vi "界面UI.vi"() -> ()   [LabVIEW 2016, in "德润DR803L超标留样.lvlib"]
uses:
  <vilib>/Utility/miscctls.llb/LVPointTypeDef.ctl
  <vilib>/Utility/config.llb/NI_LVConfig.lvlib
  <vilib>/ptbypt/NI_PtbyPt.lvlib
panel:
  in  "超标浓度配置":bool
  out "流程中":bool
  in  "停止流程":bool
  in  "启动流程":bool
  in  "时间等比采样":u16=10
  in  "单次采样量":u16=500
  in  "修改门禁密码":bool
  in  "远程复位":bool
  in  "排空当前瓶":bool
  in  "采样方式":enum16{"单采", "双重"}(ring)
  in  "远程留样":bool
  in  "选择留样瓶":bool
  in  "排空留样瓶":bool
  out "采样器状态":T1
  out "Registers":u16[](array[numeric])
  in  "打开串口":bool
  in  "释放串口":bool
  in  "留样模式":T2(ring)=enum."外控留样"
  in  "采样启动":bool
  in  "停止命令":bool
  in  "切换采样器状态":bool
  in  "时间校准":bool
  out "source":string
  out "通讯":bool
  # "只在停止时切换有效"
  # "只在待机时切换有效"
  # "默认：500ml（5-1000）ml （只在停止时写有效）"
  # "只在待机时启动有效"
  # "默认：10min（2-9999）min （只在停止时写有效）"
  # "只在待机时启动有效"
  # "只在待机时启动有效"
  # "德润DR803L超标留样"
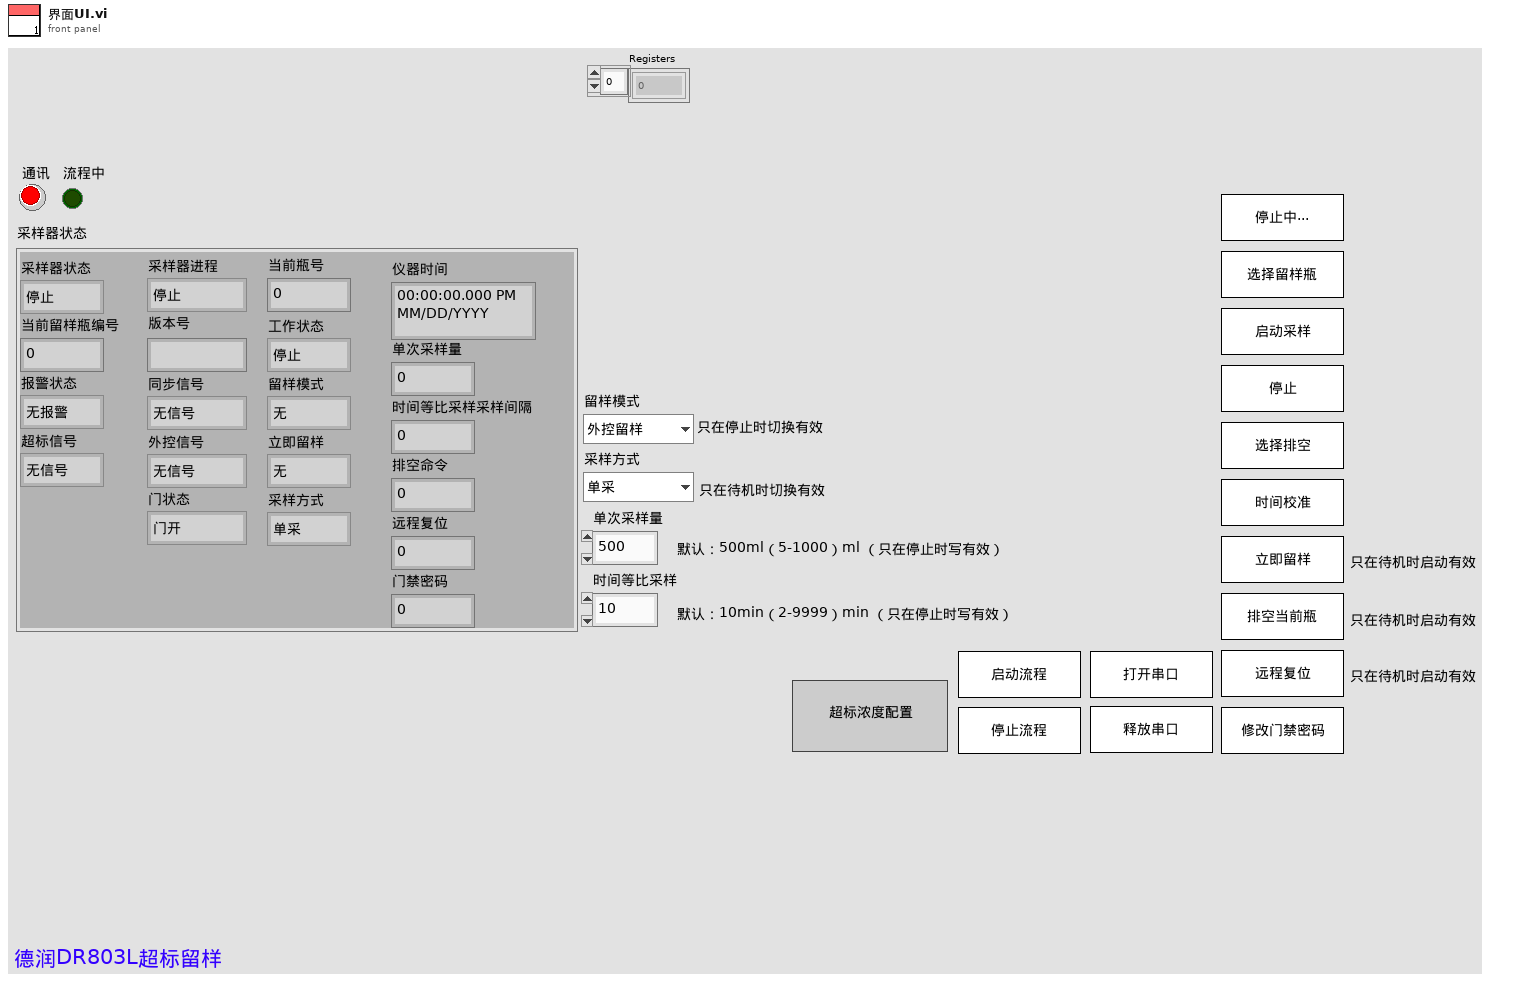
[diagram p1: front panel]
types:
  T1 = cluster{"采样器状态":enum16{"停止", "运行"}, "当前留样瓶编号":u16, "报警状态":enum16{"无报警", "缺水报警"}, "超标信号":enum16{"无信号", "超标信号"}, "采样器进程":enum16{"停止", "待机", "定位校正", "移除瓶盖", "采样瓶排空", "管路润洗", "管存", "进样", "瓶盖密封", "管路排空", "调整采样位置", "采样结束", "采样瓶润洗", "瓶润洗排空"}, "版本号":string, "同步信号":enum16{"无信号", "同步信号"}, "外控信号":enum16{"无信号", "外控信号"}, "门状态":enum16{"门开", "门关"}, "当前瓶号":u16, "工作状态":enum16{"停止", "采样中"}, "留样模式":enum16{"无", "定时留样", "时间等比例", "超标留样", "同步留样", "外控留样"}, "立即留样":enum16{"无", "远程留样"}, "采样方式":enum16{"单采", "双重"}, "仪器时间":timestamp, "单次采样量":u16, "时间等比采样采样间隔":u16, "排空命令":u16, "远程复位":u16, "门禁密码":u16}
  T2 = enum16{"无", "定时留样", "时间等比例", "超标留样", "同步留样", "外控留样"}
  T3 = cluster{"STEP":enum16{"open", "read", "write", "write single", "close"}, "starting address":u16, "value":u16}
  T4 = typedef "LVPointTypeDef.ctl" = cluster{"Horizontal":i16, "Vertical":i16}
  T5 = typedef "NI_LVConfig.lvlib/Config Data RefNum.ctl" = refnum<k1>
  T6 = enum16{"open", "read", "write", "write single", "close"}
  T7 = cluster{"氨氮超标浓度":dbl, "总磷超标浓度":dbl, "总氮超标浓度":dbl, "CODMn超标浓度":dbl, "CODCr超标浓度":dbl}
  T8 = typedef "LVDateTimeRec.ctl" = cluster{"秒数的小数部分":dbl, "秒":i32, "分":i32, "时":i32, "日":i32, "月":i32, "年":i32, "天数（周）":i32, "天数（年）":i32, "DST":i32}
  T9 = enum32{"Bad", "Idle", "Run top level", "Running"}
  T10 = cluster{"确定":bool, "氨氮超标浓度":dbl, "总磷超标浓度":dbl, "总氮超标浓度":dbl, "CODMn超标浓度":dbl, "CODCr超标浓度":dbl}
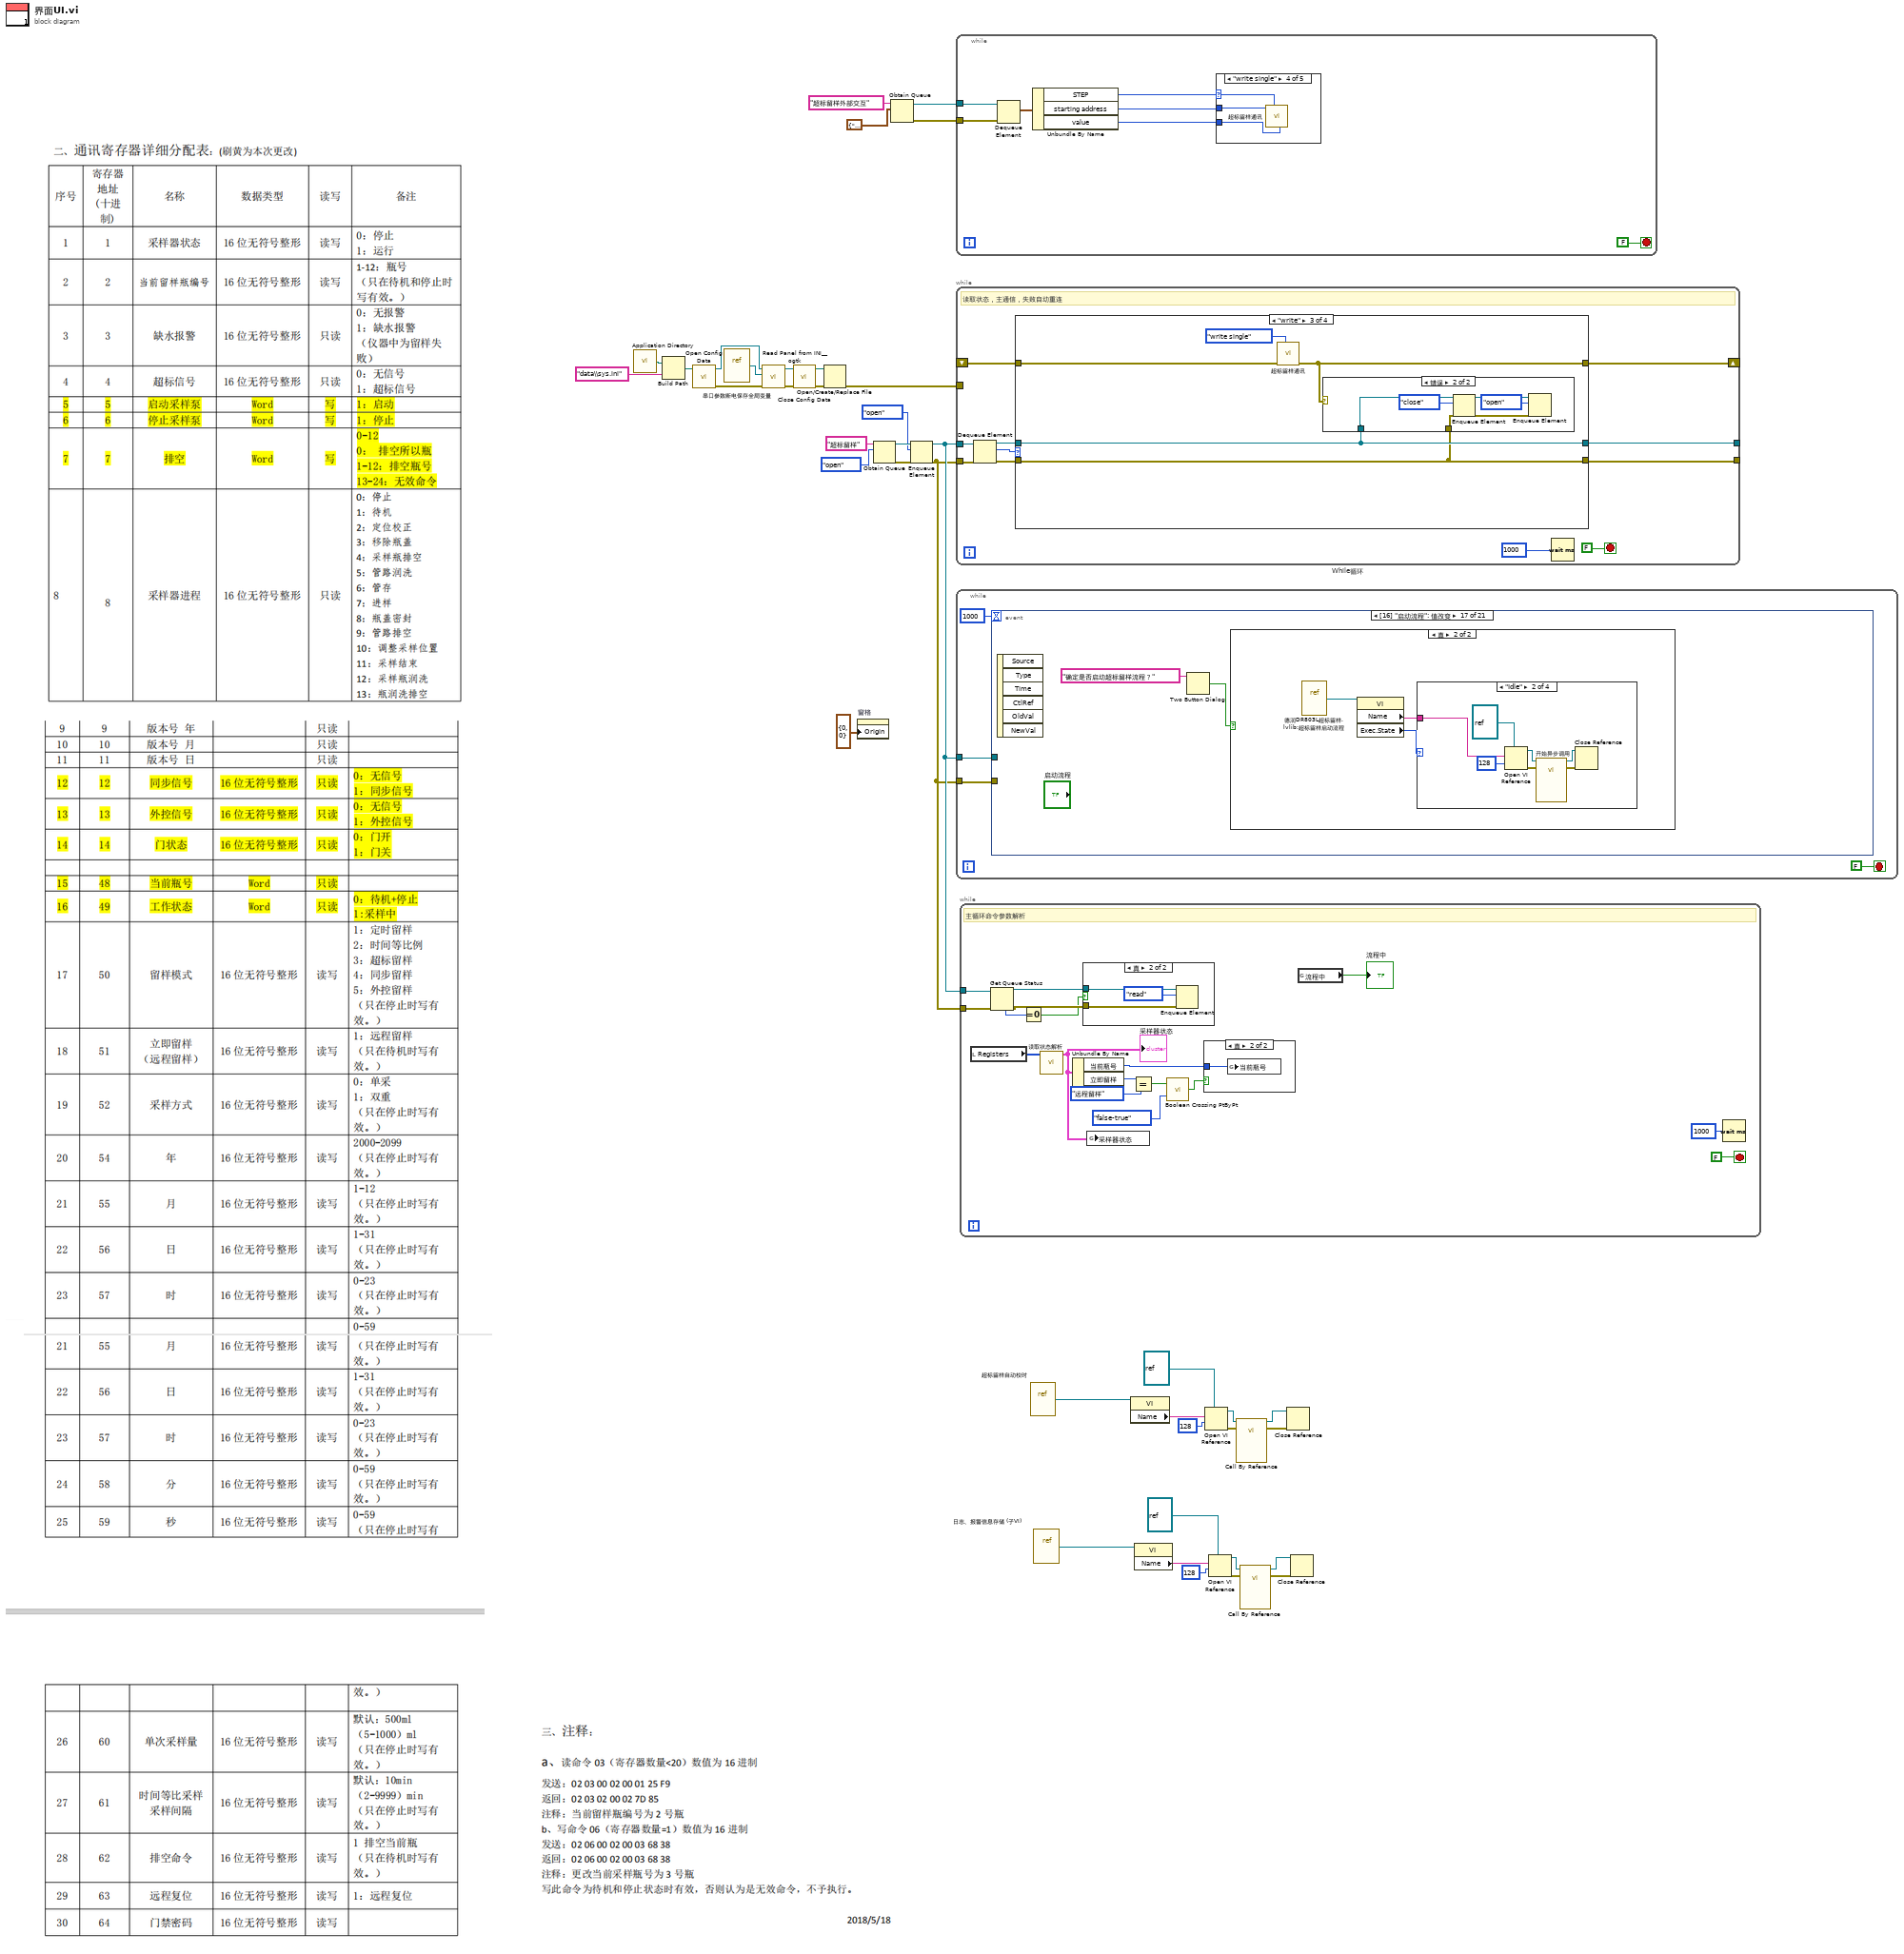
[diagram p0: block diagram]
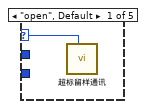
[diagram p2: hidden frame]
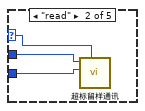
[diagram p3: hidden frame]
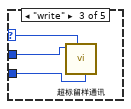
[diagram p4: hidden frame]
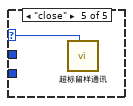
[diagram p5: hidden frame]
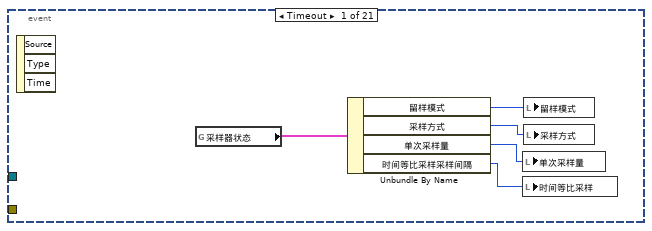
[diagram p6: hidden frame]
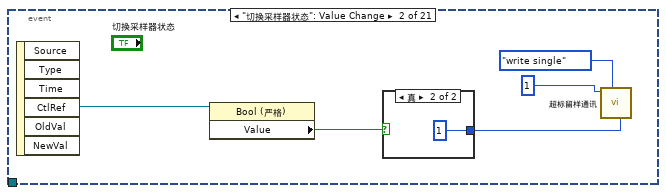
[diagram p7: hidden frame]
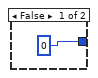
[diagram p8: hidden frame]
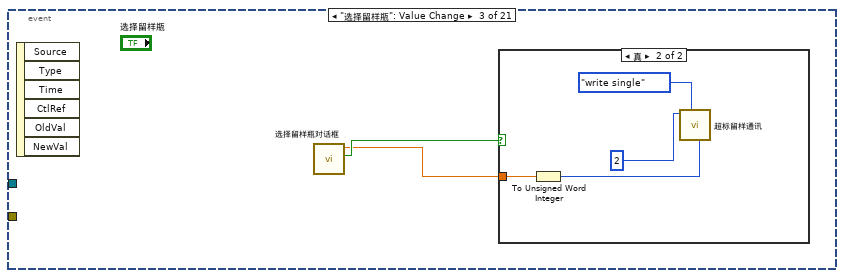
[diagram p9: hidden frame]
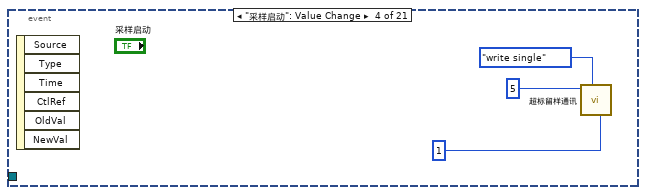
[diagram p11: hidden frame]
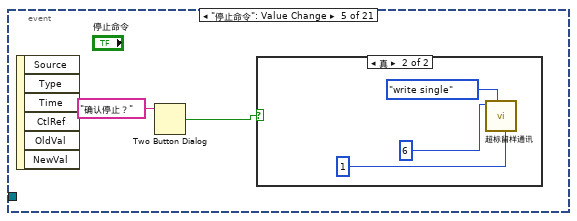
[diagram p12: hidden frame]
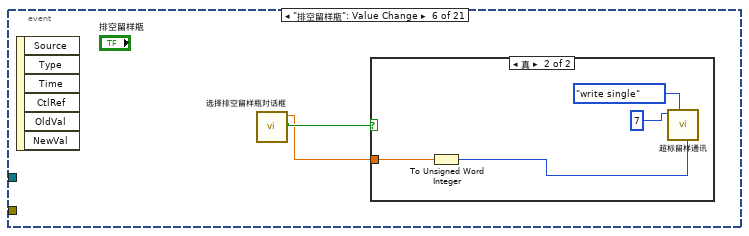
[diagram p14: hidden frame]
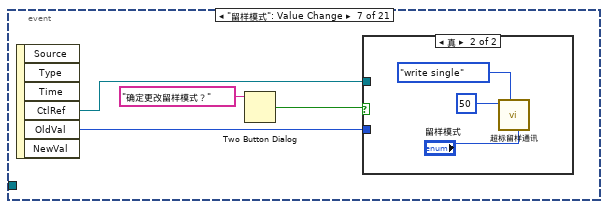
[diagram p16: hidden frame]
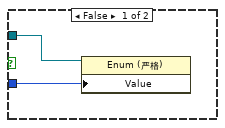
[diagram p17: hidden frame]
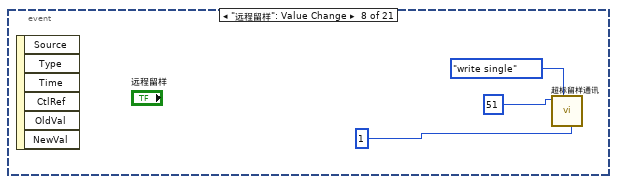
[diagram p18: hidden frame]
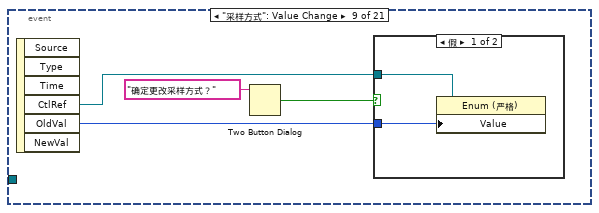
[diagram p19: hidden frame]
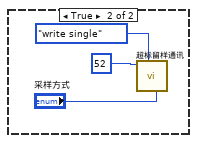
[diagram p20: hidden frame]
diagram:
  n1 = call <vilib>:"Application Directory.vi"() -> ("Application Directory"=w31:path)
  n2 = Build Path(base path=w31, name or relative path="data\\sys.ini" ("名称或相对路径")) -> (appended path=w29:path)
  n3 = call <vilib>:"Open Config Data.vi"("configuration file path"=w29) -> ("error out"=w25:errorcluster, "refnum"=w28:T5)  [unwired: 8 in, 1 out]
  n4 = vi-ref "串口参数断电保存全局变量.vi"() -> (w27:refnum<vi>)
  n5 = call <userlib>:"Read Panel from INI__ogtk.vi"("error in (no error)"=w25, "VI ref"=w27, "refnum"=w28) -> ("error out"=w24:errorcluster, "refnum out"=w26:T5)  [unwired: 7 in]
  n6 = call <vilib>:"Close Config Data.vi"("error in (no error)"=w24, "refnum"=w26) -> ("error out"=w23:errorcluster, "file path"=w22:path)  [unwired: 8 in]
  n7 = Open/Create/Replace File(file path (use dialog)=w22, error in=w23) -> (error out=w21:errorcluster)  [unwired: 4 in, 2 out]
  n8 = property on="窗格" class="Pane"("Origin"=T4 {"Horizontal"=0, "Vertical"=0} ("原点")) -> ()  [unwired: 2 in, 2 out]
  n9 = Obtain Queue(name (unnamed)="超标留样" ("名称（未命名）"), element data type=enum16{"open", "read", "write", "close"}."open") -> (queue out=w37:refnum<queue>, error out=w36:errorcluster)  [unwired: 3 in, 1 out]
  n10 = Obtain Queue(name (unnamed)="超标留样外部交互" ("名称（未命名）"), element data type=T3 {"STEP"=enum."write single", "starting address"=0, "value"=0}) -> (queue out=w18:refnum<queue>, error out=w17:errorcluster)  [unwired: 3 in, 1 out]
  n11 = Enqueue Element(queue=w37, element=enum16{"open", "read", "write", "close"}."open", error in (no error)=w36) -> (queue out=w34:refnum<queue>, error out=w33:errorcluster)  [unwired: 1 in, 1 out]
  n12 = while {
    tunnel: w34 -> [w42]
    tunnel: w33 -> [w41]
    stop <- FALSE stop-if-true
    n13 = event shown="[16] \"启动流程\": 值改变" {
      selector: _ -> [_ _ _ _ _ _ _ _ _ _ _ _ _ _ _ _ _ _ _ _ _]
      dyn-events: _ -> [_ _ _ _ _ _ _ _ _ _ _ _ _ _ _ _ _ _ _ _ _]
      timeout: 1000 -> [_ _ _ _ _ _ _ _ _ _ _ _ _ _ _ _ _ _ _ _ _]
      tunnel: w42 -> [_ _ _ _ _ _ _ _ _ _ _ _ _ _ _ _ _ _ w171 w177 _]
      tunnel: w41 -> [_ _ _ _ _ _ _ _ _ _ _ _ _ _ _ _ _ _ w170 w176 _]
      event Timeout {
        n14 = event-data() -> ()  [unwired: 1 in, 3 out]
        n15 = global read "超标留样全局.vi" "采样器状态"() -> (w44:T1)
        n16 = Unbundle By Name(w44) -> ("留样模式"=w48:T2, "采样方式"=w45:enum16{"单采", "双重"}, "单次采样量"=w46:u16, "时间等比采样采样间隔"=w47:u16)
        n17 = local write "单次采样量"(w46) -> ()
        n18 = local write "时间等比采样"(w47) -> ()
        n19 = local write "留样模式"(w48) -> ()
        n20 = local write "采样方式"(w45) -> ()
      }
      event "切换采样器状态": Value Change {
        n21 = event-data() -> ("CtlRef"=w53:refnum<vi>)  [unwired: 1 in, 5 out]
        n22 = property class="Bool (严格)"(reference=w53) -> ("Value"=w52:bool)  [unwired: 1 in, 2 out]
        n23 = case shown="真" w52 {
          tunnel: [u16 0 ("索引") u16 1 ("索引")] -> w49
          frame False {
          }
          frame True {
          }
        }
        n24 = call "超标留样通讯.vi"("value"=w49, "STEP"=T6."write single", "starting address"=1 ("索引")) -> ()  [unwired: 6 in, 3 out]
      }
      event "选择留样瓶": Value Change {
        n25 = event-data() -> ()  [unwired: 1 in, 6 out]
        n26 = call "选择留样瓶对话框.vi"() -> ("布尔"=w57:bool, "选择留样瓶"=w56:dbl)  [unwired: 10 in]
        n27 = case shown="真" w57 {
          tunnel: w56 -> [_ w58]
          frame False {
          }
          frame True {
            n28 = To Unsigned Word Integer(number=w58) -> (unsigned 16bit integer=w59:u16)
            n29 = call "超标留样通讯.vi"("value"=w59, "STEP"=T6."write single", "starting address"=2 ("索引")) -> ()  [unwired: 6 in, 3 out]
          }
        }
      }
      event "采样启动": Value Change {
        n30 = event-data() -> ()  [unwired: 1 in, 6 out]
        n31 = call "超标留样通讯.vi"("value"=u16 1 ("新元素/子数组"), "STEP"=T6."write single", "starting address"=5 ("索引")) -> ()  [unwired: 6 in, 3 out]
      }
      event "停止命令": Value Change {
        n32 = event-data() -> ()  [unwired: 1 in, 6 out]
        n33 = Two Button Dialog(message="确认停止？" ("消息")) -> (T button?=w65:bool)  [unwired: 2 in]
        n34 = case shown="真" w65 {
          frame False {
          }
          frame True {
            n35 = call "超标留样通讯.vi"("value"=u16 1 ("新元素/子数组"), "STEP"=T6."write single", "starting address"=6 ("索引")) -> ()  [unwired: 6 in, 3 out]
          }
        }
      }
      event "排空留样瓶": Value Change {
        n36 = event-data() -> ()  [unwired: 1 in, 6 out]
        n37 = call "选择排空留样瓶对话框.vi"() -> ("布尔"=w71:bool, "选择留样瓶"=w70:dbl)  [unwired: 10 in]
        n38 = case shown="真" w71 {
          tunnel: w70 -> [_ w75]
          frame False {
          }
          frame True {
            n39 = To Unsigned Word Integer(number=w75) -> (unsigned 16bit integer=w72:u16)
            n40 = call "超标留样通讯.vi"("value"=w72, "STEP"=T6."write single", "starting address"=7 ("索引")) -> ()  [unwired: 6 in, 3 out]
          }
        }
      }
      event "留样模式": Value Change {
        n41 = event-data() -> ("CtlRef"=w76:refnum<vi>, "OldVal"=w77:T2)  [unwired: 1 in, 4 out]
        n42 = Two Button Dialog(message="确定更改留样模式？" ("消息")) -> (T button?=w78:bool)  [unwired: 2 in]
        n43 = case shown="真" w78 {
          tunnel: w77 -> [w80 _]
          tunnel: w76 -> [w81 _]
          frame False {
            n44 = property class="Enum (严格)"(reference=w81, "Value"=w80) -> ()  [unwired: 1 in, 2 out]
          }
          frame True {
            n45 = call "超标留样通讯.vi"("value"="留样模式", "STEP"=T6."write single", "starting address"=50 ("索引")) -> ()  [unwired: 6 in, 3 out]
          }
        }
      }
      event "远程留样": Value Change {
        n46 = event-data() -> ()  [unwired: 1 in, 6 out]
        n47 = call "超标留样通讯.vi"("value"=u16 1 ("新元素/子数组"), "STEP"=T6."write single", "starting address"=51 ("索引")) -> ()  [unwired: 6 in, 3 out]
      }
      event "采样方式": Value Change {
        n48 = event-data() -> ("CtlRef"=w89:refnum<vi>, "OldVal"=w88:enum16{"单采", "双重"})  [unwired: 1 in, 4 out]
        n49 = Two Button Dialog(message="确定更改采样方式？" ("消息")) -> (T button?=w90:bool)  [unwired: 2 in]
        n50 = case shown="假" w90 {
          tunnel: w89 -> [w93 _]
          tunnel: w88 -> [w92 _]
          frame False {
            n51 = property class="Enum (严格)"(reference=w93, "Value"=w92) -> ()  [unwired: 1 in, 2 out]
          }
          frame True {
            n52 = call "超标留样通讯.vi"("value"="采样方式", "STEP"=T6."write single", "starting address"=52 ("索引")) -> ()  [unwired: 6 in, 3 out]
          }
        }
      }
      event "时间校准": Value Change {
        n53 = event-data() -> ()  [unwired: 1 in, 6 out]
        n54 = Get Date/Time In Seconds() -> (seconds since 1Jan1904=w109:timestamp)
        n55 = Seconds To Date/Time(time stamp (now)=w109) -> (date time rec=w108:T8)  [unwired: 1 in]
        n56 = Unbundle By Name(w108) -> ("年"=w105:i32, "月"=w104:i32, "日"=w103:i32, "时"=w102:i32, "分"=w101:i32, "秒"=w100:i32)
        n57 = Build Array(w105, w104, w103, w102, w101, w100) -> (w99:i32[])
        n58 = Insert Into Array(array=u16[] [] ("values"), new element=w99) -> (w106:u16[])  [unwired: 1 in]
        n59 = call "超标留样通讯.vi"("STEP"=T6."write", "values"=w106, "starting address"=54 ("索引")) -> ()  [unwired: 6 in, 3 out]
      }
      event "单次采样量", "时间等比采样": Mouse Down {
        n60 = event-data() -> ("CtlRef"=w113:refnum<vi>)  [unwired: 1 in, 7 out]
        n61 = property class="DigNum (严格)"(reference=w113) -> (reference out=w112:refnum<vi>, "Value"=w111:u16)  [unwired: 1 in, 1 out]
        n62 = call "数字键盘.vi"("OldNumber"=w111) -> ("NewNumber"=w110:sgl)
        n63 = property class="DigNum (严格)"(reference=w112, "Val(Sgnl)"=w110) -> ()  [unwired: 1 in, 2 out]
      }
      event "单次采样量": Value Change {
        n64 = event-data() -> ()  [unwired: 1 in, 6 out]
        n65 = call "超标留样通讯.vi"("value"="单次采样量", "STEP"=T6."write single", "starting address"=60 ("索引")) -> ()  [unwired: 6 in, 3 out]
      }
      event "时间等比采样": Value Change {
        n66 = event-data() -> ()  [unwired: 1 in, 6 out]
        n67 = call "超标留样通讯.vi"("value"="时间等比采样", "STEP"=T6."write single", "starting address"=61 ("索引")) -> ()  [unwired: 6 in, 3 out]
      }
      event "排空当前瓶": Value Change {
        n68 = event-data() -> ()  [unwired: 1 in, 6 out]
        n69 = Two Button Dialog(message="是否排空当前瓶？" ("消息")) -> (T button?=w120:bool)  [unwired: 2 in]
        n70 = case shown="真" w120 {
          frame False {
          }
          frame True {
            n71 = call "超标留样通讯.vi"("value"=u16 1 ("新元素/子数组"), "STEP"=T6."write single", "starting address"=63 ("索引")) -> ()  [unwired: 6 in, 3 out]
          }
        }
      }
      event "远程复位": Value Change {
        n72 = event-data() -> ()  [unwired: 1 in, 6 out]
        n73 = Two Button Dialog(message="确认复位？" ("消息")) -> (T button?=w125:bool)  [unwired: 2 in]
        n74 = case shown="真" w125 {
          frame False {
          }
          frame True {
            n75 = call "超标留样通讯.vi"("value"=u16 1 ("新元素/子数组"), "STEP"=T6."write single", "starting address"=64 ("索引")) -> ()  [unwired: 6 in, 3 out]
          }
        }
      }
      event "修改门禁密码": Value Change {
        n76 = event-data() -> ()  [unwired: 1 in, 6 out]
        n77 = Two Button Dialog(message="确定修改门禁密码？" ("消息")) -> (T button?=w130:bool)  [unwired: 2 in]
        n78 = case shown="真" w130 {
          frame False {
          }
          frame True {
            n79 = local read "采样器状态"() -> (w133:T1)
            n80 = Unbundle By Name(w133) -> ("门禁密码"=w132:u16)
            n81 = call "数字键盘.vi"("OldNumber"=w132) -> ("NewNumber"=w136:sgl)
            n82 = Less?(x=w136, y=sgl 65535.0) -> (x < y?=w134:bool)
            n83 = case shown="真" w134 {
              tunnel: w136 -> [_ w140]
              frame False {
              }
              frame True {
                n84 = To Unsigned Word Integer(number=w140) -> (unsigned 16bit integer=w137:u16)
                n85 = call "超标留样通讯.vi"("value"=w137, "STEP"=T6."write single", "starting address"=65 ("索引")) -> ()  [unwired: 6 in, 3 out]
              }
            }
          }
        }
      }
      event "启动流程": Value Change {
        n86 = event-data() -> ()  [unwired: 1 in, 6 out]
        n87 = Two Button Dialog(message="确定是否启动超标留样流程？" ("消息")) -> (T button?=w141:bool)  [unwired: 2 in]
        n88 = case shown="真" w141 {
          frame False {
          }
          frame True {
            n89 = vi-ref "德润DR803L超标留样.lvlib:超标留样启动流程.vi"() -> (w143:refnum<vi>)
            n90 = property class="VI"(reference=w143) -> ("Name"=w144:string, "Exec.State"=w145:T9)  [unwired: 1 in, 2 out]
            n91 = case shown="\"Idle\"" w145 {
              tunnel: w144 -> [_ w148 _ _]
              frame "Bad", Default {
              }
              frame "Idle" {
                n92 = Open VI Reference(type specifier VI Refnum (for type only)=refnum<vi> refnum ("类型说明符VI引用句柄（仅用于类型）"), vi path=w148, options=128 ("选项")) -> (vi reference=w152:refnum<vi>, error out=w147:errorcluster)  [unwired: 3 in]
                n93 = call-by-ref "开始异步调用"(reference=w152, error in=w147) -> (reference out=w151:refnum<vi>, error out=w146:errorcluster)  [unwired: 12 in]
                n94 = Close Reference(reference=w151, error in (no error)=w146) -> ()  [unwired: 1 out]
              }
              frame "Run top level" {
              }
              frame "Running" {
              }
            }
          }
        }
      }
      event "停止流程": Value Change {
        n95 = event-data() -> ()  [unwired: 1 in, 6 out]
        n96 = Two Button Dialog(message="确定是否停止超标留样流程并排空当前瓶？" ("消息")) -> (T button?=w153:bool)  [unwired: 2 in]
        n97 = case shown="真" w153 {
          frame False {
          }
          frame True {
            n98 = Obtain Notifier(name (unnamed)="超标留样流程" ("名称（未命名）"), notification data type=FALSE ("采样完成")) -> (notifier out=w166:refnum<notifier>, error out=w165:errorcluster)  [unwired: 2 in, 1 out]
            n99 = Send Notification(notification=TRUE ("通知"), notifier=w166, error in (no error)=w165) -> (notifier out=w163:refnum<notifier>, error out=w162:errorcluster)
            n100 = call "超标留样通讯.vi"("value"=u16 1 ("新元素/子数组"), "STEP"=T6."write single", "starting address"=6 ("索引")) -> ("error out"=w155:errorcluster)  [unwired: 6 in, 2 out]
            n101 = Release Notifier(notifier=w163, error in (no error)=w162) -> ()  [unwired: 1 in, 3 out]
            n102 = call "超标留样通讯.vi"("value"=u16 1 ("新元素/子数组"), "STEP"=T6."write single", "Error in"=w155, "starting address"=63 ("索引")) -> ()  [unwired: 5 in, 3 out]
          }
        }
      }
      event "释放串口": Value Change {
        n103 = event-data() -> ()  [unwired: 1 in, 6 out]
        n104 = Two Button Dialog(message="确认是否释放串口，释放串口将导致通信失败！" ("消息")) -> (T button?=w169:bool)  [unwired: 2 in]
        n105 = case shown="真" w169 {
          tunnel: w171 -> [_ w174]
          tunnel: w170 -> [_ w173]
          frame False {
          }
          frame True {
            n106 = Enqueue Element(queue=w174, element=enum16{"open", "read", "write", "close"}."close" ("元素"), error in (no error)=w173) -> ()  [unwired: 1 in, 3 out]
          }
        }
      }
      event "打开串口": Value Change {
        n107 = event-data() -> ()  [unwired: 1 in, 6 out]
        n108 = global read "串口参数断电保存全局变量.vi" "VISA resource name"() -> (w185:refnum<visa-resource-name>)
        n109 = global read "串口参数断电保存全局变量.vi" "MB通信方式选择"() -> (w186:enum16{"串口", "TCP"})
        n110 = global read "串口参数断电保存全局变量.vi" "PORT"() -> (w183:string)
        n111 = global read "串口参数断电保存全局变量.vi" "IP"() -> (w184:string)
        n112 = call "串口配置.vi"("PORT"=w183, "IP"=w184, "MB通信方式选择"=w186, "请选择串口:"=w185) -> ("PORT 2"=w179:string, "IP 2"=w180:string, "确认 2"=w182:bool, "VISA资源名称 2"=w181:refnum<visa-resource-name>, "MB通信方式选择 2"=w178:enum16{"串口", "TCP"})  [unwired: 3 in]
        n113 = case shown="真" w182 {
          tunnel: w181 -> [_ w194]
          tunnel: w180 -> [_ w193]
          tunnel: w179 -> [_ w192]
          tunnel: w178 -> [_ w191]
          tunnel: w177 -> [_ w190]
          tunnel: w176 -> [_ w188]
          frame False {
          }
          frame True {
            n114 = flat-sequence {
              tunnel: w194 -> [w200]
              tunnel: w193 -> [w199]
              tunnel: w192 -> [w198]
              tunnel: w191 -> [w197]
              tunnel: w190 -> [w196]
              tunnel: [w196] -> w189
              tunnel: w188 -> [w195]
              tunnel: [w195] -> w187
              tunnel: w189 -> [w202]
              tunnel: w187 -> [w201]
              frame #0 {
                n115 = global write "串口参数断电保存全局变量.vi" "VISA resource name"(w200) -> ()
                n116 = global write "串口参数断电保存全局变量.vi" "MB通信方式选择"(w197) -> ()
                n117 = global write "串口参数断电保存全局变量.vi" "PORT"(w198) -> ()
                n118 = global write "串口参数断电保存全局变量.vi" "IP"(w199) -> ()
              }
              frame #1 {
                n119 = call <vilib>:"Application Directory.vi"() -> ("Application Directory"=w205:path)
                n120 = Build Path(base path=w205, name or relative path="data\\sys.ini" ("名称或相对路径")) -> (appended path=w206:path)
                n121 = Enqueue Element(queue=w202, element=enum16{"open", "read", "write", "close"}."open" ("元素"), error in (no error)=w201) -> ()  [unwired: 1 in, 3 out]
                n122 = call <vilib>:"Open Config Data.vi"("configuration file path"=w206) -> ("error out"=w210:errorcluster, "refnum"=w207:T5)  [unwired: 8 in, 1 out]
                n123 = vi-ref "串口参数断电保存全局变量.vi"() -> (w208:refnum<vi>)
                n124 = call <userlib>:"Write Panel to INI__ogtk.vi"("error in (no error)"=w210, "VI ref"=w208, "refnum"=w207) -> ("error out"=w211:errorcluster, "refnum out"=w209:T5)  [unwired: 7 in]
                n125 = call <vilib>:"Close Config Data.vi"("error in (no error)"=w211, "refnum"=w209) -> ("error out"=w216:errorcluster, "file path"=w217:path)  [unwired: 8 in]
                n126 = Open/Create/Replace File(file path (use dialog)=w217, error in=w216) -> (refnum out=w213:refnum<file>, error out=w212:errorcluster)  [unwired: 4 in, 1 out]
                n127 = Flush File(refnum=w213, error in=w212) -> (refnum out=w214:refnum<file>, error out=w215:errorcluster)
                n128 = Close File(refnum=w214, error in=w215) -> ()  [unwired: 2 out]
              }
            }
          }
        }
      }
      event "超标浓度配置": Value Change {
        n129 = event-data() -> ()  [unwired: 1 in, 6 out]
        n130 = global read "串口参数断电保存全局变量.vi" "CODMn超标浓度"() -> (w229:dbl)
        n131 = global read "串口参数断电保存全局变量.vi" "CODCr超标浓度"() -> (w228:dbl)
        n132 = global read "串口参数断电保存全局变量.vi" "总磷超标浓度"() -> (w226:dbl)
        n133 = global read "串口参数断电保存全局变量.vi" "总氮超标浓度"() -> (w230:dbl)
        n134 = global read "串口参数断电保存全局变量.vi" "氨氮超标浓度"() -> (w227:dbl)
        n135 = Bundle By Name(cluster=T7 {"氨氮超标浓度"=0.0, "总磷超标浓度"=0.0, "总氮超标浓度"=0.0, "CODMn超标浓度"=0.0, "CODCr超标浓度"=0.0} ("输入"), "氨氮超标浓度"=w227, "总磷超标浓度"=w226, "总氮超标浓度"=w230, "CODMn超标浓度"=w229, "CODCr超标浓度"=w228) -> (w225:T7)
        n136 = call "超标浓度设置.vi"("输入"=w225) -> ("输出"=w224:T10)  [unwired: 10 in]
        n137 = Unbundle By Name(w224) -> ("确定"=w223:bool, "氨氮超标浓度"=w222:dbl, "总磷超标浓度"=w221:dbl, "总氮超标浓度"=w220:dbl, "CODMn超标浓度"=w219:dbl, "CODCr超标浓度"=w218:dbl)
        n138 = case shown="真" w223 {
          tunnel: w222 -> [_ w236]
          tunnel: w221 -> [_ w235]
          tunnel: w220 -> [_ w234]
          tunnel: w219 -> [_ w233]
          tunnel: w218 -> [_ w232]
          frame False {
          }
          frame True {
            n139 = flat-sequence {
              tunnel: w236 -> [w241]
              tunnel: w235 -> [w240]
              tunnel: w234 -> [w239]
              tunnel: w233 -> [w238]
              tunnel: w232 -> [w237]
              frame #0 {
                n140 = global write "串口参数断电保存全局变量.vi" "CODMn超标浓度"(w238) -> ()
                n141 = global write "串口参数断电保存全局变量.vi" "CODCr超标浓度"(w237) -> ()
                n142 = global write "串口参数断电保存全局变量.vi" "总磷超标浓度"(w240) -> ()
                n143 = global write "串口参数断电保存全局变量.vi" "总氮超标浓度"(w239) -> ()
                n144 = global write "串口参数断电保存全局变量.vi" "氨氮超标浓度"(w241) -> ()
              }
              frame #1 {
                n145 = call <vilib>:"Application Directory.vi"() -> ("Application Directory"=w243:path)
                n146 = Build Path(base path=w243, name or relative path="data\\sys.ini" ("名称或相对路径")) -> (appended path=w244:path)
                n147 = call <vilib>:"Open Config Data.vi"("configuration file path"=w244) -> ("error out"=w248:errorcluster, "refnum"=w245:T5)  [unwired: 8 in, 1 out]
                n148 = vi-ref "串口参数断电保存全局变量.vi"() -> (w246:refnum<vi>)
                n149 = call <userlib>:"Write Panel to INI__ogtk.vi"("error in (no error)"=w248, "VI ref"=w246, "refnum"=w245) -> ("error out"=w249:errorcluster, "refnum out"=w247:T5)  [unwired: 7 in]
                n150 = call <vilib>:"Close Config Data.vi"("error in (no error)"=w249, "refnum"=w247) -> ("error out"=w254:errorcluster, "file path"=w255:path)  [unwired: 8 in]
                n151 = Open/Create/Replace File(file path (use dialog)=w255, error in=w254) -> (refnum out=w251:refnum<file>, error out=w250:errorcluster)  [unwired: 4 in, 1 out]
                n152 = Flush File(refnum=w251, error in=w250) -> (refnum out=w252:refnum<file>, error out=w253:errorcluster)
                n153 = Close File(refnum=w252, error in=w253) -> ()  [unwired: 2 out]
              }
            }
          }
        }
      }
    }
  }
  n154 = while {
    tunnel: w18 -> [w261]
    tunnel: w17 -> [w260]
    stop <- FALSE stop-if-true
    n155 = Dequeue Element(queue=w261, error in (no error)=w260) -> (element=w259:T3)  [unwired: 1 in, 3 out]
    n156 = Unbundle By Name(w259) -> ("STEP"=w258:T6, "starting address"=w257:u16, "value"=w256:u16)
    n157 = case shown="\"write single\"" w258 {
      selector: w258 -> [w263 w266 w269 w272 w273]
      tunnel: w257 -> [_ w265 w268 w271 _]
      tunnel: w256 -> [_ w264 w267 w270 _]
      frame "open", Default {
        n158 = call "超标留样通讯.vi"("STEP"=w263) -> ()  [unwired: 8 in, 3 out]
      }
      frame "read" {
        n159 = call "超标留样通讯.vi"("STEP"=w266, "quantity"=w264, "starting address"=w265) -> ()  [unwired: 6 in, 3 out]
      }
      frame "write" {
        n160 = call "超标留样通讯.vi"("value"=w267, "STEP"=w269, "starting address"=w268) -> ()  [unwired: 6 in, 3 out]
      }
      frame "write single" {
        n161 = call "超标留样通讯.vi"("value"=w270, "STEP"=w272, "starting address"=w271) -> ()  [unwired: 6 in, 3 out]
      }
      frame "close" {
        n162 = call "超标留样通讯.vi"("STEP"=w273) -> ()  [unwired: 8 in, 3 out]
      }
    }
  }
  n163 = while "While循环" {
    tunnel: w34 -> [w275]
    tunnel: w33 -> [w274]
    tunnel: [w279] -> _
    tunnel: [w278] -> _
    shift-right: [w276] -> _
    shift-left: _ -> [w277]
    tunnel: w21 -> [_]
    stop <- FALSE stop-if-true
    # "读取状态，主通信，失败自动重连"
    n164 = Dequeue Element(queue=w275, error in (no error)=w274) -> (queue out=w281:refnum<queue>, element=w282:enum16{"open", "read", "write", "close"}, error out=w280:errorcluster)  [unwired: 1 in, 1 out]
    n165 = case shown="\"write\"" w282 {
      tunnel: [w290 w292 w311 w320] -> w276
      tunnel: w281 -> [w289 w296 w310 w323]
      tunnel: w280 -> [w288 w295 w309 w322]
      tunnel: [w289 w296 w310 w323] -> w279
      tunnel: [w288 w295 w309 w322] -> w278
      tunnel: w277 -> [w287 w301 w313 w324]
      frame "open", Default {
        n166 = call "超标留样通讯.vi"("STEP"=T6."open", "Error in"=w287) -> ("error out"=w290:errorcluster, "MB session in"=w286:refnum<class "MB_Master.lvclass">)  [unwired: 7 in, 1 out]
        n167 = global write "串口参数断电保存全局变量.vi" "MB session in"(w286) -> ()
      }
      frame "read" {
        n168 = call "超标留样通讯.vi"("STEP"=T6."read", "Error in"=w301, "quantity"=u16 70, "starting address"=u16 0) -> ("error out"=w292:errorcluster, "Registers"=w298:u16[])  [unwired: 5 in, 1 out]
        n169 = Unbundle By Name(w292) -> ("status"=w294:bool, "source"=→"source":string)
        n170 = Not(x=w294) -> (.not. x?=w291:bool)
        "通讯" <- w291
        n171 = global write "超标留样全局.vi" "通讯"(w291) -> ()
        n172 = case shown="无错误" w292 {
          tunnel: w298 -> [w302 _]
          tunnel: w296 -> [_ w307]
          tunnel: w295 -> [_ w306]
          frame No Error {
            "Registers" <- w302
          }
          frame Error {
            n173 = Enqueue Element(queue=w307, element=enum16{"open", "read", "write", "close"}."close" ("元素"), error in (no error)=w306) -> (queue out=w305:refnum<queue>, error out=w304:errorcluster)  [unwired: 1 in, 1 out]
            n174 = Enqueue Element(queue=w305, element=enum16{"open", "read", "write", "close"}."open" ("元素"), error in (no error)=w304) -> ()  [unwired: 1 in, 3 out]
          }
        }
      }
      frame "write" {
        n175 = call "超标留样通讯.vi"("STEP"=T6."write single", "Error in"=w313) -> ("error out"=w311:errorcluster)  [unwired: 7 in, 2 out]
        n176 = case shown="错误" w311 {
          tunnel: w310 -> [_ w315]
          tunnel: w309 -> [_ w314]
          frame No Error {
          }
          frame Error {
            n177 = Enqueue Element(queue=w315, element=enum16{"open", "read", "write", "close"}."close" ("元素"), error in (no error)=w314) -> (queue out=w318:refnum<queue>, error out=w317:errorcluster)  [unwired: 1 in, 1 out]
            n178 = Enqueue Element(queue=w318, element=enum16{"open", "read", "write", "close"}."open" ("元素"), error in (no error)=w317) -> ()  [unwired: 1 in, 3 out]
          }
        }
      }
      frame "close" {
        n179 = call "超标留样通讯.vi"("STEP"=T6."close", "Error in"=w324) -> ("error out"=w320:errorcluster)  [unwired: 7 in, 2 out]
      }
    }
    n180 = Wait (ms)(milliseconds to wait=u32 1000 ("等待时间（毫秒）")) -> ()  [unwired: 1 out]
  }
  n181 = while {
    tunnel: w34 -> [w339]
    tunnel: w33 -> [w338]
    stop <- FALSE stop-if-true
    # "主循环命令参数解析"
    n182 = local read "Registers"() -> (w333:u16[])
    n183 = Get Queue Status(queue=w339, error in (no error)=w338) -> (queue out=w336:refnum<queue>, error out=w335:errorcluster, # elements in queue=w337:i32)  [unwired: 1 in, 5 out]
    n184 = Equal To 0?(x=w337) -> (x = 0?=w334:bool)
    n185 = call "读取状态解析.vi"("Registers"=w333) -> ("采样器状态"=w326:T1)  [unwired: 9 in, 1 out]
    "采样器状态" <- w326
    n186 = Unbundle By Name(w326) -> ("当前瓶号"=w328:u16, "立即留样"=w332:enum16{"无", "远程留样"})
    n187 = case shown="真" w334 {
      tunnel: w336 -> [_ w344]
      tunnel: w335 -> [_ w343]
      frame False {
      }
      frame True {
        n188 = Enqueue Element(queue=w344, element=enum16{"open", "read", "write", "close"}."read" ("元素"), error in (no error)=w343) -> ()  [unwired: 1 in, 3 out]
      }
    }
    n189 = global write "超标留样全局.vi" "采样器状态"(w326) -> ()
    n190 = Equal?(x=w332, y=enum16{"无", "远程留样"}."远程留样") -> (x = y?=w331:bool)
    n191 = call <vilib>:"Boolean Crossing PtByPt.vi"("direction"=enum16{"either", "false-true", "true-false"}."false-true", "input"=w331) -> ("crossing"=w329:bool)  [unwired: 1 in]
    n192 = case shown="真" w329 {
      tunnel: w328 -> [_ w342]
      frame False {
      }
      frame True {
        n193 = global write "超标留样全局.vi" "当前瓶号"(w342) -> ()
      }
    }
    n194 = global read "串口参数断电保存全局变量.vi" "流程中"() -> (→"流程中":bool)
    n195 = Wait (ms)(milliseconds to wait=u32 1000 ("等待时间（毫秒）")) -> ()  [unwired: 1 out]
  }
  n196 = vi-ref "超标留样自动校时.vi"() -> (w8:refnum<vi>)
  n197 = vi-ref "日志、报警信息存储 (子VI).vi"() -> (w9:refnum<vi>)
  n198 = property class="VI"(reference=w8) -> ("Name"=w7:string)  [unwired: 1 in, 2 out]
  n199 = property class="VI"(reference=w9) -> ("Name"=w10:string)  [unwired: 1 in, 2 out]
  n200 = Open VI Reference(type specifier VI Refnum (for type only)=refnum<vi> refnum, vi path=w7, options=128 ("选项")) -> (vi reference=w5:refnum<vi>, error out=w3:errorcluster)  [unwired: 3 in]
  n201 = Open VI Reference(type specifier VI Refnum (for type only)=refnum<vi> refnum, vi path=w10, options=128 ("选项")) -> (vi reference=w12:refnum<vi>, error out=w14:errorcluster)  [unwired: 3 in]
  n202 = call-by-ref "?"(reference=w5, error in=w3) -> (reference out=w1:refnum<vi>, error out=w2:errorcluster)  [unwired: 12 in]
  n203 = call-by-ref "?"(reference=w12, error in=w14) -> (reference out=w16:refnum<vi>, error out=w15:errorcluster)  [unwired: 12 in]
  n204 = Close Reference(reference=w1, error in (no error)=w2) -> ()  [unwired: 1 out]
  n205 = Close Reference(reference=w16, error in (no error)=w15) -> ()  [unwired: 1 out]
